vi "MathcadV.vi"() -> ()   [LabVIEW 2010]
uses:
  ADT 2/Variable cluster.ctl
  <vilib>/Utility/file.llb/Write To Spreadsheet File (string).vi
  ADT 2/AguaClara Library.lvlib
panel:
  in  "ReFresh File":bool
  out "Variable Clusters out":T1
  out "Full Names":string[][](array[string])
  in  "Save to XLS":bool
  out "XML":string
  in  "Find Variables":bool
  in  "stop":bool
  in  "Path":path
  # "Select a single file"
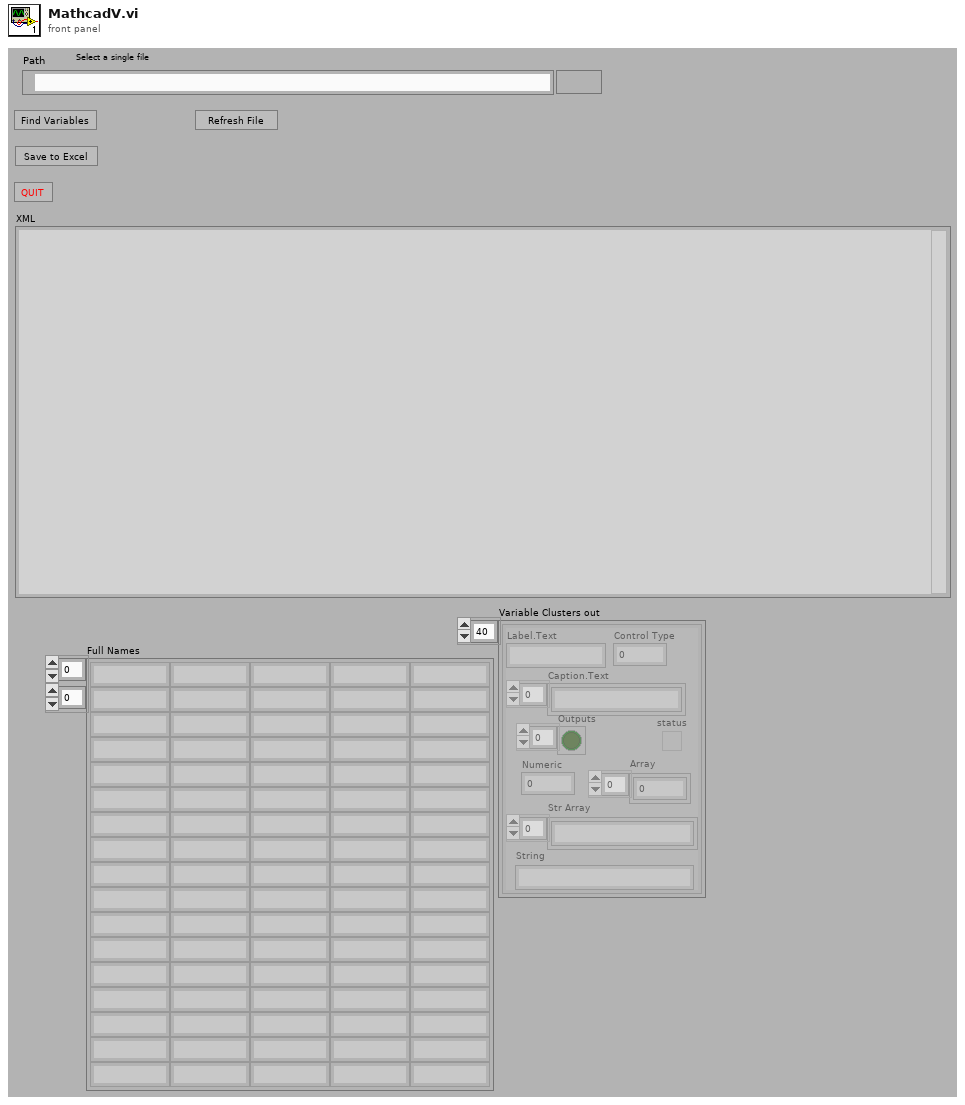
[diagram p1: front panel]
types:
  T1 = typedef "Variable cluster.ctl" = cluster{"Label.Text":string, "Caption.Text":string[], "Control Type":u32, "Numeric":dbl, "Array":dbl[], "status":bool, "Outputs":bool[], "Str Array":string[], "String":string}[]
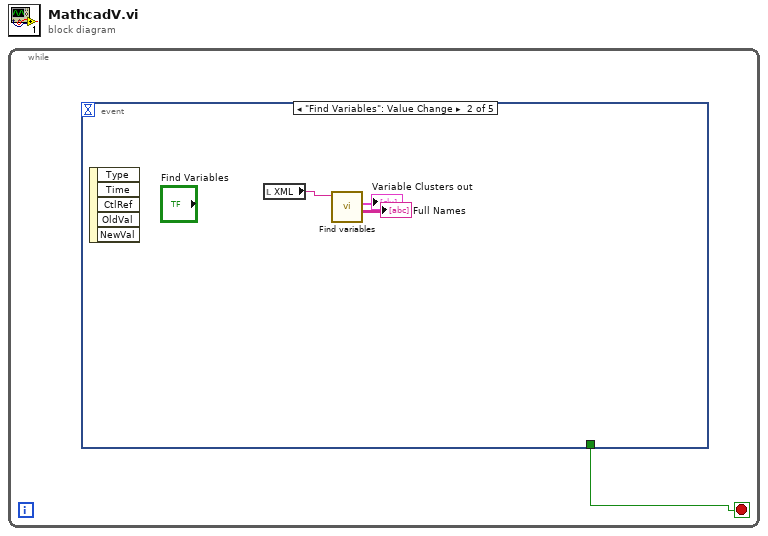
[diagram p0: block diagram]
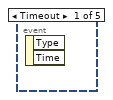
[diagram p2: hidden frame]
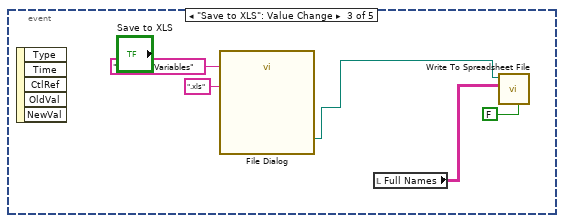
[diagram p3: hidden frame]
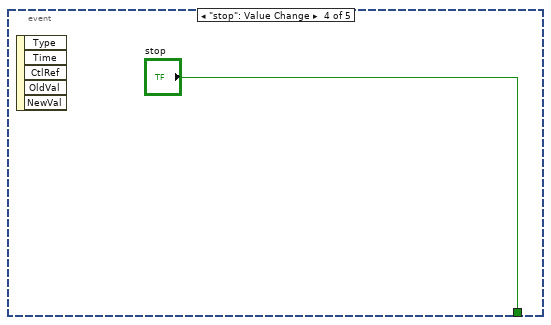
[diagram p4: hidden frame]
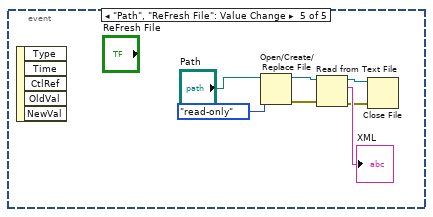
[diagram p5: hidden frame]
diagram:
  n1 = while {
    stop <- w1 stop-if-true
    n2 = event shown="[1] \"Find Variables\": Value Change" {
      selector: _ -> [_ _ _ _ _]
      dyn-events: _ -> [_ _ _ _ _]
      timeout: _ -> [_ _ _ _ _]
      tunnel: [_ _ _ "stop" _] -> w1
      event Timeout {
        n3 = event-data() -> ()  [unwired: 1 in, 2 out]
      }
      event "Find Variables": Value Change {
        n4 = event-data() -> ()  [unwired: 1 in, 5 out]
        n5 = local read "XML"() -> (w4:string)
        n6 = call "Find variables.vi"("XML"=w4) -> ("Full Names"=→"Full Names":string[][], "Variable Clusters out"=→"Variable Clusters out":T1)  [unwired: 8 in, 1 out]
      }
      event "Save to XLS": Value Change {
        n7 = event-data() -> ()  [unwired: 1 in, 5 out]
        n8 = call "File Dialog"("default name"="Mathcad Variables", "pattern (all files)"=".xls") -> ("selected path"=w6:path)  [unwired: 10 in, 3 out]
        n9 = local read "Full Names"() -> (w5:string[][])
        n10 = call-poly <vilib>:"Write To Spreadsheet File.vi"("transpose? (no:F)"=FALSE, "2D data"=w5, "file path (dialog if empty)"=w6) -> ()  [unwired: 5 in, 1 out]
      }
      event "stop": Value Change {
        n11 = event-data() -> ()  [unwired: 1 in, 5 out]
      }
      event "Path", "ReFresh File": Value Change {
        n12 = event-data() -> ()  [unwired: 1 in, 5 out]
        n13 = Open/Create/Replace File(file path (use dialog)="Path", access (0:read/write)=enum16{"read/write", "read-only", "write-only"}."read-only") -> (refnum out=w15:refnum<file>, error out=w16:errorcluster)  [unwired: 4 in, 1 out]
        n14 = Read from Text File(file (use dialog)=w15, error in=w16) -> (refnum out=w12:refnum<file>, text=→"XML":string, error out=w11:errorcluster)  [unwired: 2 in, 1 out]
        n15 = Close File(refnum=w12, error in=w11) -> ()  [unwired: 2 out]
      }
    }
  }
